vi "Close Queues.vi"(8 "error in (no error)":errorcluster, 11 "FIFOs In":T1) -> (0 "error out":errorcluster)   [LabVIEW 2020, in "Queues.lvlib"]
doc: "Copyright 2015, 2016, 2017 National Instruments Corporation\n\nLicensed under the Apache License, Version 2.0 (the \"License\"); you may not use this file except in compliance with the License.\n\n You may obtain a copy of the License at\n\n http://www.apache.org/licenses/LICENSE-2.0\n\nUnless required by applicable law or agreed to in writing, software distributed under the License is distributed on an \"AS IS\" BASIS, WITHOUT WARRANTIES OR CONDITIONS OF ANY KIND, either express or implied.\n\nSee the License for the specific language governing permissions and limitations under the License."
uses:
  Queues.lvlib
  Queue Refs.ctl
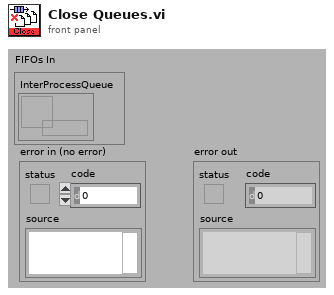
[diagram p1: front panel]
types:
  T1 = typedef "Queues.lvlib/Queue Refs.ctl" = cluster{"InterProcessQueue":refnum<queue>}
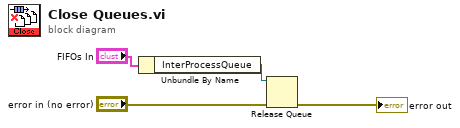
[diagram p0: block diagram]
diagram:
  n1 = Unbundle By Name("FIFOs In") -> ("InterProcessQueue"=w3:refnum<queue>)
  n2 = Release Queue(queue=w3, error in (no error)="error in (no error)") -> (error out=→"error out":errorcluster)  [unwired: 3 out]
